vi "Send NI prepare task.vi"(7 "Message Priority (Normal)":T2=enum."Normal", 8 "error in (no error)":errorcluster, 10 "NI task parameters":T1, 11 "Message Enqueuer":refnum<class "Message Enqueuer.lvclass">) -> (0 "error out":errorcluster, 3 "Message Enqueuer out":refnum<class "Message Enqueuer.lvclass">)   [LabVIEW 2021, in "NI.lvlib" / "NI prepare task Msg.lvclass"]
doc: "This VI sends the message to an actor."
uses:
  NI prepare task Msg.lvclass
  <vilib>/ActorFramework/Message Enqueuer/Message Enqueuer.lvclass
  <vilib>/ActorFramework/Message Enqueuer/Message Priority.ctl
  NI/NI task parameters.ctl
  C:/Program Files (x86)/National Instruments/LabVIEW 2021/vi.lib/ActorFramework/Message/Message.lvclass
  NI prepare task Msg.lvclass/NI prepare task Msg.ctl
  <vilib>/ActorFramework/Message Enqueuer/Message Enqueuer.lvclass/Message Enqueuer.ctl
  <vilib>/ActorFramework/Message Priority Queue/Priority Enqueue.vi
  NI/NI.lvclass
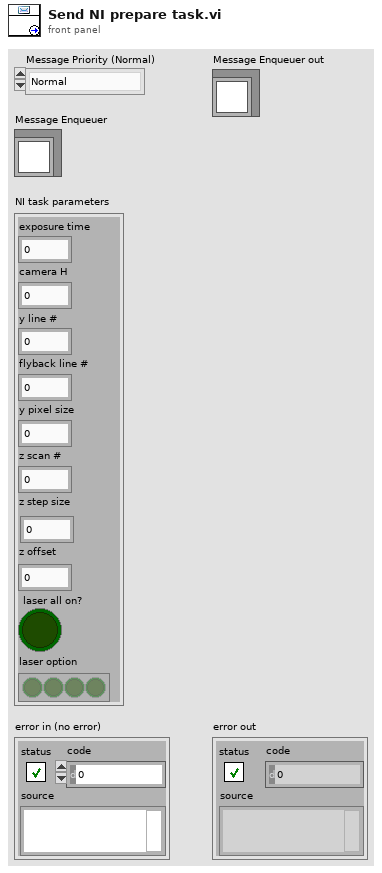
[diagram p1: front panel]
types:
  T1 = typedef "NI.lvlib/NI.lvclass/NI task parameters.ctl" = cluster{"exposure time":dbl, "camera H":dbl, "y line #":dbl, "flyback line #":dbl, "y pixel size":dbl, "z scan #":dbl, "z step size":dbl, "z offset":dbl, "laser all on?":bool, "laser option":bool[]}
  T2 = typedef "Actor Framework.lvlib/Message Enqueuer.lvclass/Message Priority.ctl" = enum16{"Low", "Normal", "High"}
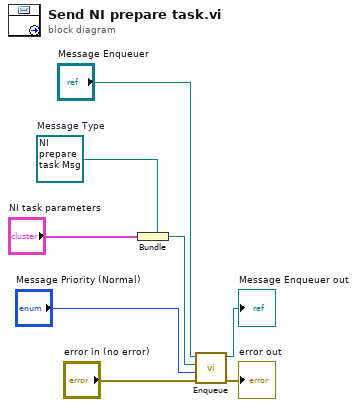
[diagram p0: block diagram]
diagram:
  w5 = refnum<class "NI prepare task Msg.lvclass"> refnum  # Message Type
  n1 = Bundle(cluster=w5, "NI task parameters") -> (w4:refnum<class "NI prepare task Msg.lvclass">)
  n2 = call <vilib>:"Enqueue.vi"("error in (no error)"="error in (no error)", "Message Priority (Normal)"="Message Priority (Normal)", "Message"=w4, "Message Enqueuer in"="Message Enqueuer") -> ("error out"=→"error out":errorcluster, "Message Enqueuer out"=→"Message Enqueuer out":refnum<class "Message Enqueuer.lvclass">)  [unwired: 6 in]
